vi "SC_schleife_init_mischer.vi"() -> ()   [LabVIEW 2019]
uses:
  Global/Global Variables/global.vi
  Global/Global Variables/Data_Display_global.vi
  Instrument_Setup.vi
panel:
  out "Numeric 3":dbl format="%#_13g"
  out "Numeric 2":dbl format="%#_13g"
  out "XY Graph":T1(graph)
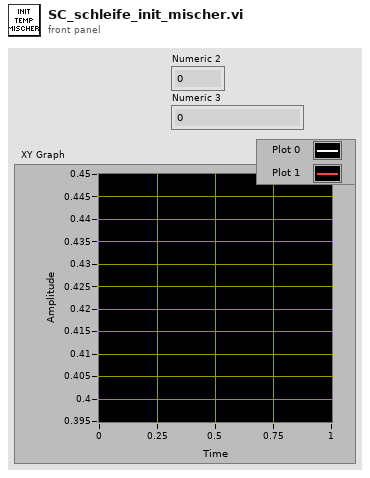
[diagram p1: front panel]
types:
  T1 = cluster{"Plot1":dbl[], "Best Linear Fit":dbl[]}[]
  T2 = typedef "LS372-Cluster.ctl" = cluster{"Activate Tsweep":bool, "Setpoint - Manual":dbl, "Rate (K/min)":dbl, "Update Lakeshores":bool, "Still Heater":bool, "Still Power (mW)":dbl, "Manual Heater":bool, "Manual Heater  (mW) ":dbl, "Heater Range":dbl, "P (Gain)":dbl, "I (Reset)":dbl, "D (Rate)":dbl, "Heater Power (mW)":dbl, "MC Thermometer":u16, "MC Temperature":dbl, "LS372-T1":dbl, "LS372 -T2":dbl, "LS372-R1 ":dbl, "LS372-R2":dbl, "LS372-T3":dbl, "LS372-T4":dbl, "LS372-R3 ":dbl, "LS372-R4 \n\n\n\n":dbl, "LS372-T5":dbl, "LS372-T6":dbl, "LS372-R5":dbl, "LS372-R6 ":dbl, "Still Power ist":dbl, "Set Temperatur Sweep main":bool, "Setpoint ist":dbl, "Disable Heater":bool}
  T3 = typedef "Ls372-Control.ctl" = cluster{"Activate Tsweep":bool, "Setpoint - Manual":dbl, "Rate (K/min)":dbl, "Update Lakeshores":bool, "Still Heater":bool, "Still Power (mW)":dbl, "Manual Heater":bool, "Manual Heater  (mW) ":dbl, "MC Thermometer":u16, "Set Temperature Sweeep main":bool, "Disable Heater":bool}
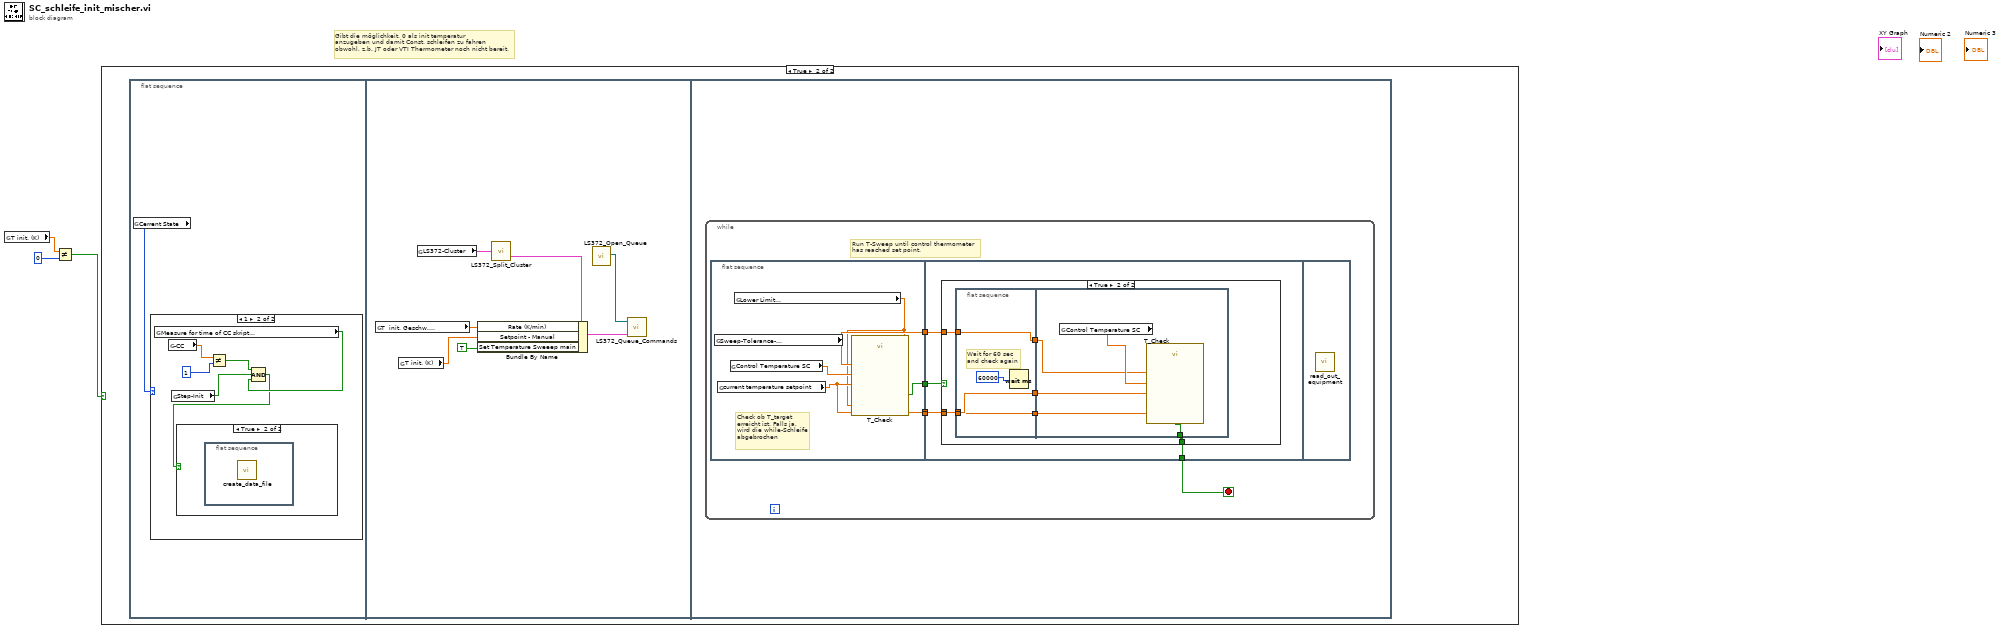
[diagram p0: block diagram]
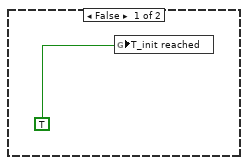
[diagram p2: hidden frame]
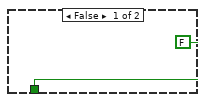
[diagram p5: hidden frame]
diagram:
  # "Gibt die möglichkeit, 0 als init temperatur \nanzugeben und damit Const. schleifen zu fahren\nobwohl, z.b. JT oder VTI Thermometer noch nicht bereit."
  n1 = global read "global.vi" "T init. (K)"() -> (w3:dbl)
  n2 = Not Equal?(x=w3, y=0) -> (x != y?=w1:bool)
  n3 = case shown="True" w1 {
    frame False {
      n4 = global write "Data_Display_global.vi" "T_init reached"(TRUE) -> ()
    }
    frame True {
      n5 = flat-sequence {
        frame #0 {
          n6 = global read "global.vi" "Cerrent State"() -> (w5:i32)
          n7 = case shown="1" w5 {
            frame 0, Default {
            }
            frame 1 {
              n8 = global read "Instrument_Setup.vi" "Measure for time of CC skript\nat each field step point"() -> (w7:bool)
              n9 = global read "global.vi" "-CC"() -> (w11:dbl)
              n10 = global read "global.vi" "Step-Init"() -> (w8:bool)
              n11 = Not Equal?(x=w11, y=1) -> (x != y?=w9:bool)
              n12 = Compound Arithmetic op=AND(w9, w8, w7) -> (w6:bool)
              n13 = case shown="True" w6 {
                frame False {
                }
                frame True {
                  n14 = flat-sequence {
                    frame #0 {
                      n15 = call "create_data_file.vi"() -> ()  [unwired: 3 in]
                    }
                  }
                }
              }
            }
          }
        }
        frame #1 {
          n16 = global read "global.vi" "T  init. Geschw. \n(K/min)"() -> (w15:dbl)
          n17 = global read "global.vi" "T init. (K)"() -> (w12:dbl)
          n18 = global read "Data_Display_global.vi" "LS372-Cluster"() -> (w18:T2)
          n19 = call "LS372_Split_Cluster.vi"("LS372-Cluster"=w18) -> ("LS372-Control"=w17:T3)  [unwired: 1 out]
          n20 = Bundle By Name(cluster=w17, "Rate (K/min)"=w15, "Setpoint - Manual"=w12, "Set Temperature Sweeep main"=TRUE) -> (w13:T3)
          n21 = call "LS372_Open_Queue.vi"() -> ("queue out"=w14:refnum<queue>)  [unwired: 10 in, 1 out]
          n22 = call "LS372_Queue_Commands.vi"("LS372-Control"=w13, "Queue"=w14) -> ()  [unwired: 1 in, 1 out]
        }
        frame #2 {
          n23 = while {
            stop <- w22 stop-if-true
            # "Run T-Sweep until control thermometer\nhas reached set point."
            n24 = flat-sequence {
              tunnel: [w27] -> w23
              tunnel: [w25] -> w21
              tunnel: [w26] -> w20
              tunnel: [w24] -> w19
              tunnel: w23 -> [w33]
              tunnel: [w32] -> w22
              tunnel: w21 -> [w31]
              tunnel: w20 -> [w30]
              tunnel: w19 -> [w29]
              frame #0 {
                # "Check ob T_target\nerreicht ist. Falls ja,\nwird die while-Schleife\nabgebrochen"
                n25 = global read "Instrument_Setup.vi" "Sweep-Tolerance-\nTemperature (%)"() -> (w26:dbl)
                n26 = global read "Data_Display_global.vi" "current temperature setpoint"() -> (w25:dbl)
                n27 = global read "Data_Display_global.vi" "Control Temperature SC"() -> (w28:dbl)
                n28 = global read "Instrument_Setup.vi" "Lower Limit\nSweep-Tolerance-\nTemperature (K)"() -> (w24:dbl)
                n29 = call "T_Check.vi"("Lower Limit Sweep\nTolerance (K)"=w24, "T_target (K)"=w25, "Sweep\nTolerance %"=w26, "T_in"=w28) -> ("= T target"=w27:bool)
              }
              frame #1 {
                n30 = case shown="True" w33 {
                  tunnel: [FALSE w41] -> w32
                  tunnel: w31 -> [_ w40]
                  tunnel: w30 -> [_ w37]
                  tunnel: w29 -> [_ w35]
                  frame False {
                  }
                  frame True {
                    n31 = flat-sequence {
                      tunnel: w40 -> [w44]
                      tunnel: [w44] -> w39
                      tunnel: [w43] -> w38
                      tunnel: w37 -> [w43]
                      tunnel: [w42] -> w36
                      tunnel: w35 -> [w42]
                      tunnel: [w50] -> w41
                      tunnel: w39 -> [w48]
                      tunnel: w38 -> [w47]
                      tunnel: w36 -> [w46]
                      frame #0 {
                        # "Wait for 60 sec\nand check again"
                        n32 = Wait (ms)(milliseconds to wait=60000) -> ()  [unwired: 1 out]
                      }
                      frame #1 {
                        n33 = global read "Data_Display_global.vi" "Control Temperature SC"() -> (w49:dbl)
                        n34 = call "T_Check.vi"("Lower Limit Sweep\nTolerance (K)"=w46, "T_target (K)"=w48, "Sweep\nTolerance %"=w47, "T_in"=w49) -> ("= T target"=w50:bool)
                      }
                    }
                  }
                }
              }
              frame #2 {
                n35 = call "read_out_equipment.vi"() -> ()  [unwired: 1 in]
              }
            }
          }
        }
      }
    }
  }
